vi "Write vertical offset (0.0 V).vi"(8 "error in (no error)":errorcluster, 10 "vertical offset (0.0 V)":dbl[unit] format="%.3f", 11 "Configure Channel Msg in":refnum<class "Configure Channel Msg.lvclass">) -> (0 "error out":errorcluster, 3 "Configure Channel Msg out":refnum<class "Configure Channel Msg.lvclass">)   [LabVIEW 2016, in "CS++Scope.lvlib" / "Configure Channel Msg.lvclass"]
uses:
  Configure Channel Msg.lvclass
  Configure Channel Msg.lvclass/Configure Channel Msg.ctl
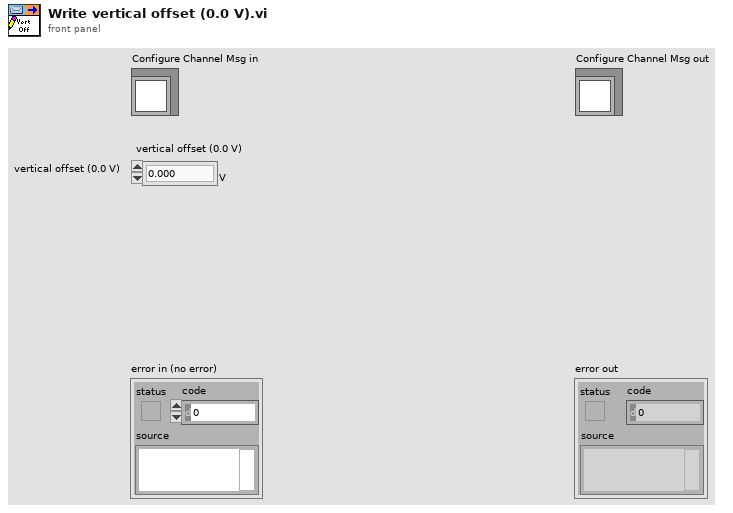
[diagram p1: front panel]
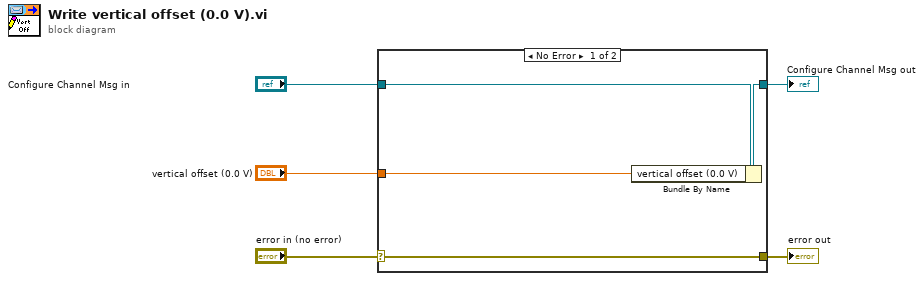
[diagram p0: block diagram]
diagram:
  n1 = case shown="No Error" "error in (no error)" {
    selector: "error in (no error)" -> [w9 w10]
    tunnel: [w9 w10] -> w4
    tunnel: [w7 w11] -> w2
    tunnel: "Configure Channel Msg in" -> [w8 w11]
    tunnel: "vertical offset (0.0 V)" -> [w6 _]
    frame No Error {
      n2 = Bundle By Name(cluster=w8, "vertical offset (0.0 V)"=w6) -> (w7:refnum<class "Configure Channel Msg.lvclass">)
    }
    frame Error {
    }
  }
  "error out" <- w4
  "Configure Channel Msg out" <- w2
